vi "Get Database Manager.vi"(8 "error in (no error)":errorcluster, 11 "Dataset in":refnum<class "Dataset.lvclass">) -> (0 "error out":errorcluster, 2 "Database Manager":refnum<class "Database Manager.lvclass">, 3 "Dataset out":refnum<class "Dataset.lvclass">)   [LabVIEW 2019, in "HierDAL Library.lvlib" / "Database.lvlib" / "Repositories.lvlib" / "Dataset.lvclass"]
uses:
  Dataset.lvclass
  Database Manager Class/Database Manager.lvclass
  Dataset.lvclass/Dataset.ctl
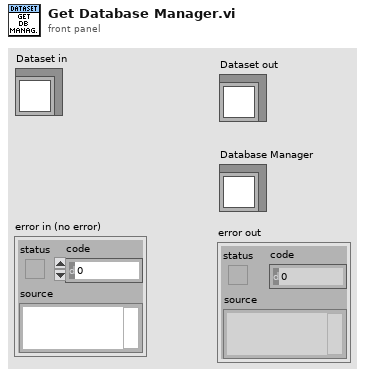
[diagram p1: front panel]
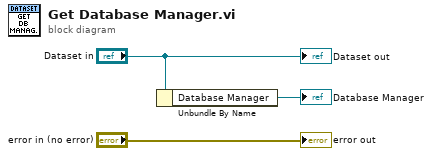
[diagram p0: block diagram]
diagram:
  n1 = Unbundle By Name("Dataset in") -> ("Database Manager"=→"Database Manager":refnum<class "Database Manager.lvclass">)
  "error out" <- "error in (no error)"
  "Dataset out" <- "Dataset in"
